vi "Repack Pixels_Pixel Bus to FIFO U8x8.vi"(10 "Input Valid":bool=TRUE, 11 "Pixel Bus In":T1={"Pixel Data"=[0, 0, 0, 0, 0, 0, 0, 0], "DV"=[FALSE, FALSE, FALSE, FALSE, FALSE, FALSE, FALSE, FALSE], "EOL"=FALSE, "EOI"=FALSE, "Data Type"=enum."U8 x 8"}) -> (2 "Output Valid":bool, 3 "output array":u8[](array[numeric]))   [LabVIEW 2020, in "NI_VDM_FPGA_Basics.lvlib"]
uses:
  <vilib>/visionFPGA/NI_VDM_FPGA_Basics.lvlib
  <vilib>/visionFPGA/Controls/IMAQ FPGA Pixel Bus u8x8.ctl
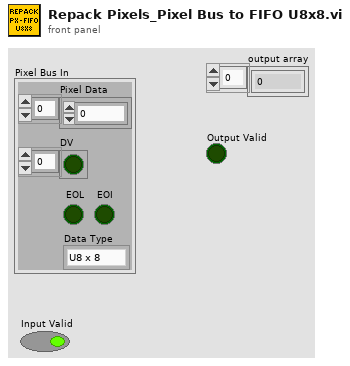
[diagram p1: front panel]
types:
  T1 = typedef "IMAQ FPGA Pixel Bus u8x8.ctl" = cluster{"Pixel Data":u8[], "DV":bool[], "EOL":bool, "EOI":bool, "Data Type":enum16{"U8 x 8"}}
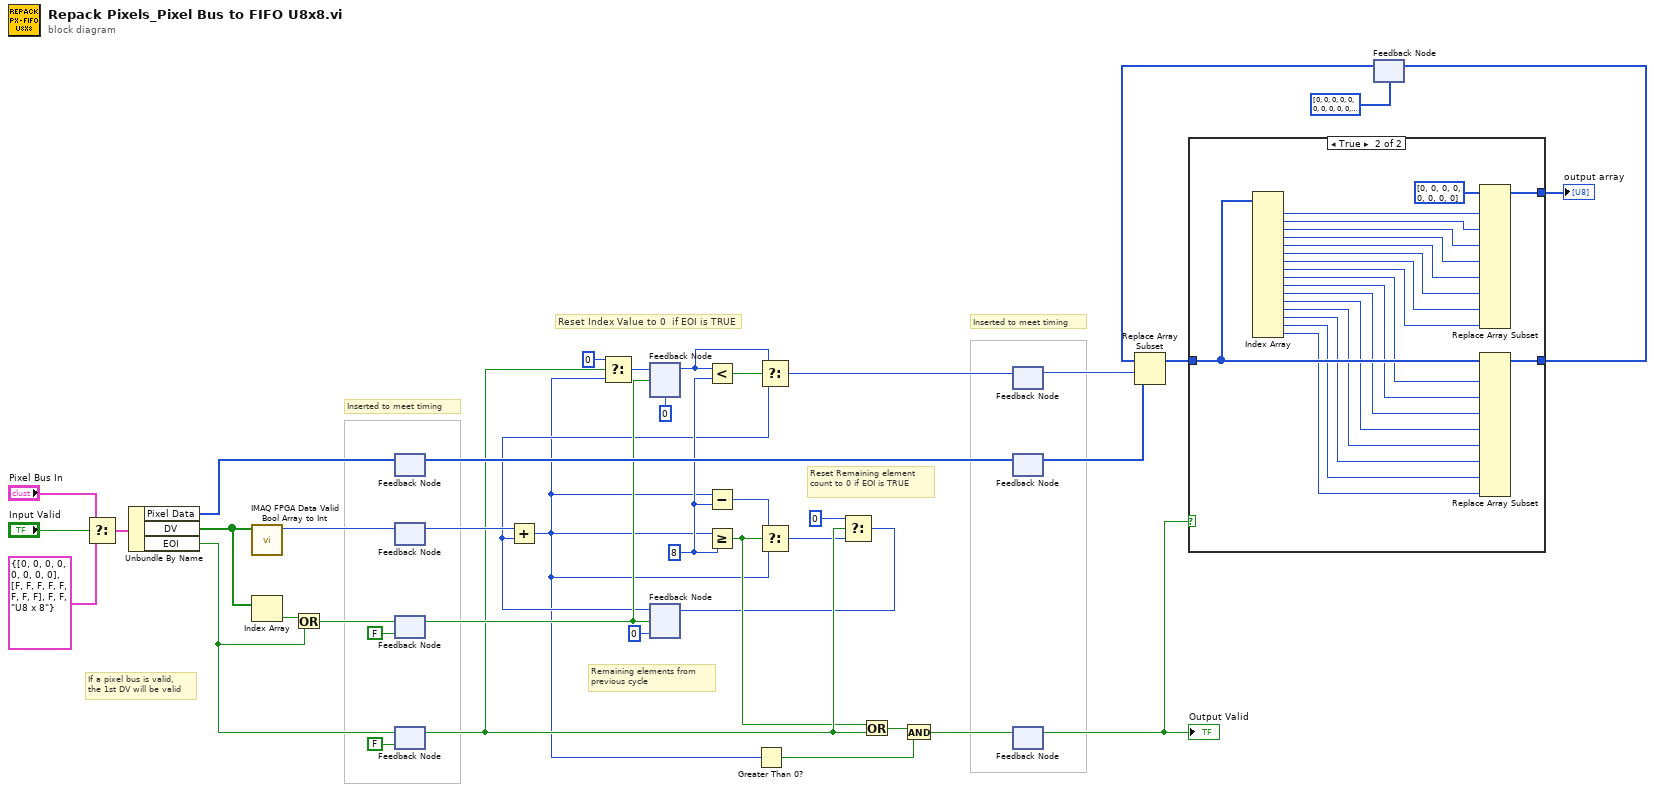
[diagram p0: block diagram]
diagram:
  w22 = u16 8 ("y")
  # "If a pixel bus is valid,\nthe 1st DV will be valid"
  # "Inserted to meet timing"
  # "Inserted to meet timing"
  # "Reset Remaining element count to 0 if EOI is TRUE"
  # "Reset Index Value to 0  if EOI is TRUE"
  # "Remaining elements from \nprevious cycle"
  n1 = Select(t="Pixel Bus In", s="Input Valid", f=T1 {"Pixel Data"=[0, 0, 0, 0, 0, 0, 0, 0], "DV"=[FALSE, FALSE, FALSE, FALSE, FALSE, FALSE, FALSE, FALSE], "EOL"=FALSE, "EOI"=FALSE, "Data Type"=enum."U8 x 8"}) -> (s? t:f=w38:T1)
  n2 = Unbundle By Name(w38) -> ("Pixel Data"=w37:u8[], "DV"=w2:bool[], "EOI"=w31:bool)
  n3 = call <vilib>:"IMAQ FPGA Data Valid Bool Array to Int.vi"("DV In"=w2) -> ("Sum DV Out"=w35:u8)  [unwired: 10 in]
  n4 = Index Array(array=w2) -> (element=w1:bool)  [unwired: 1 in]
  n5 = Or(x=w1, y=w31) -> (x .or. y?=w33:bool)
  n6 = feedback-in #1(w37) -> ()
  n7 = feedback #1() -> (w36:u8[])  [unwired: 1 in]
  n8 = feedback #2() -> (w34:u8)  [unwired: 1 in]
  n9 = feedback-in #2(w35) -> ()
  n10 = feedback #3(FALSE) -> (w32:bool)
  n11 = feedback-in #3(w33) -> ()
  n12 = feedback #4(FALSE ("EOI")) -> (w30:bool)
  n13 = feedback-in #4(w31) -> ()
  n14 = feedback #5(u16 0 ("t")) -> (w21:u16)
  n15 = feedback #6(u16 0 ("t")) -> (w18:u16)
  n16 = Add(x=w34, y=w18) -> (x+y=w11:u16)
  n17 = Select(t=u16 0, s=w30, f=w11) -> (s? t:f=w13:u16)
  n18 = feedback-in #5(w13, w32) -> ()
  n19 = Less?(x=w21, y=w22) -> (x < y?=w20:bool)
  n20 = Subtract(x=w11, y=w22) -> (x-y=w23:u16)
  n21 = Greater Or Equal?(x=w11, y=w22) -> (x >= y?=w19:bool)
  n22 = Greater Than 0?(x=w11) -> (x > 0?=w10:bool)
  n23 = Select(t=w21, s=w20, f=w18) -> (s? t:f=w9:u16)
  n24 = Select(t=w23, s=w19, f=w11) -> (s? t:f=w16:u16)
  n25 = Select(t=u16 0, s=w30, f=w16) -> (s? t:f=w14:u16)
  n26 = feedback-in #6(w14, w32) -> ()
  n27 = Or(x=w19, y=w30) -> (x .or. y?=w17:bool)
  n28 = And(x=w17, y=w10) -> (x .and. y?=w6:bool)
  n29 = feedback #7() -> (w8:u16)  [unwired: 1 in]
  n30 = feedback-in #7(w9) -> ()
  n31 = feedback #8() -> (w7:u8[])  [unwired: 1 in]
  n32 = feedback-in #8(w36) -> ()
  n33 = feedback #9() -> (w41:bool)  [unwired: 1 in]
  "Output Valid" <- w41
  n34 = feedback-in #9(w6) -> ()
  n35 = feedback #10(u8[] [0, 0, 0, 0, 0, 0, 0, 0, 0, 0, 0, 0, 0, 0, 0, 0] ("Pixel Data")) -> (w25:u8[])
  n36 = Replace Array Subset(array=w25, new element=w7, index=w8) -> (w24:u8[])
  n37 = case shown="True" w41 {
    tunnel: [w43 w63] -> w26
    tunnel: w24 -> [w43 w62]
    tunnel: [_ w44] -> w42
    frame False {
    }
    frame True {
      n38 = Index Array(array=w62) -> (element #1=w60:u8, element #2=w59:u8, element #3=w58:u8, element #4=w57:u8, element #5=w56:u8, element #6=w55:u8, element #7=w54:u8, element #8=w53:u8, element #9=w52:u8, element #10=w51:u8, element #11=w50:u8, element #12=w49:u8, element #13=w48:u8, element #14=w47:u8, element #15=w46:u8, element #16=w45:u8)  [unwired: 16 in]
      n39 = Replace Array Subset(array=u8[] [0, 0, 0, 0, 0, 0, 0, 0] ("Pixel Data"), new element #1=w60, new element #2=w59, new element #3=w58, new element #4=w57, new element #5=w56, new element #6=w55, new element #7=w54, new element #8=w53) -> (w44:u8[])  [unwired: 8 in]
      n40 = Replace Array Subset(array=w62, new element #1=w52, new element #2=w51, new element #3=w50, new element #4=w49, new element #5=w48, new element #6=w47, new element #7=w46, new element #8=w45) -> (w63:u8[])  [unwired: 8 in]
    }
  }
  "output array" <- w42
  n41 = feedback-in #10(w26) -> ()
